vi "GetMatlabBoundControlCollectionVariant.vi"(11 "ExpID":string) -> (3 "BoundControlCollectionVariant":variant)   [LabVIEW 2017]
uses:
  MatlabGlobals.vi
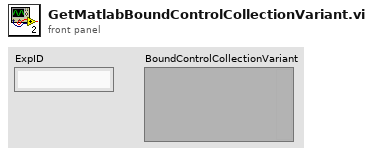
[diagram p1: front panel]
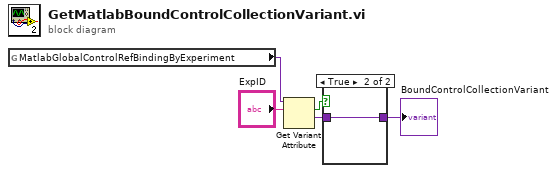
[diagram p0: block diagram]
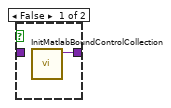
[diagram p2: hidden frame]
diagram:
  n1 = global read "MatlabGlobals.vi" "MatlabGlobalControlRefBindingByExperiment"() -> (w2:variant)
  n2 = Get Variant Attribute(Variant=w2, name="ExpID") -> (found=w4:bool, value=w1:variant)  [unwired: 2 in, 2 out]
  n3 = case shown="True" w4 {
    tunnel: w1 -> [_ w7]
    tunnel: [w6 w7] -> w5
    frame False {
      n4 = call "InitMatlabBoundControlCollection.vi"() -> ("BoundControlCollectionVariant"=w6:variant)  [unwired: 11 in]
    }
    frame True {
    }
  }
  "BoundControlCollectionVariant" <- w5
